vi "Hab Lifter TeleOp - PID.vi"(11 "Controller Values":T1) -> ()   [LabVIEW 2018]
uses:
  Support Code/Controller Values.ctl
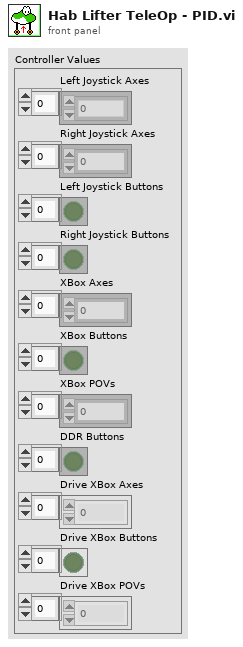
[diagram p1: front panel]
types:
  T1 = typedef "Controller Values.ctl" = cluster{"Left Joystick Axes ":dbl[], "Right Joystick Axes":dbl[], "Left Joystick Buttons":bool[], "Right Joystick Buttons":bool[], "XBox Axes":dbl[], "XBox Buttons":bool[], "XBox POVs":i16[], "DDR Buttons":bool[], "Drive XBox Axes":dbl[], "Drive XBox Buttons":bool[], "Drive XBox POVs":i16[]}
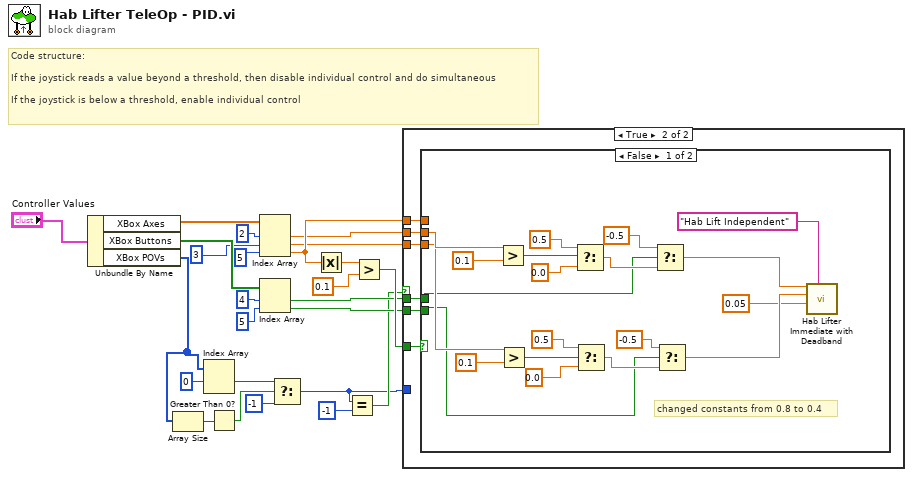
[diagram p0: block diagram]
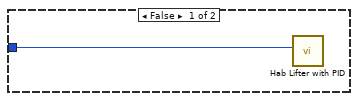
[diagram p2: hidden frame]
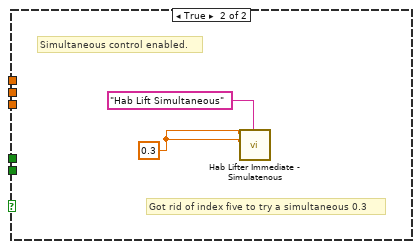
[diagram p3: hidden frame]
diagram:
  # "Code structure:\n\nIf the joystick reads a value beyond a threshold, then disable individual control and do simultaneous\n\nIf the joystick is below a threshold, enable individual control"
  n1 = Unbundle By Name("Controller Values") -> ("XBox Axes"=w24:dbl[], "XBox Buttons"=w23:bool[], "XBox POVs"=w1:i16[])
  n2 = Array Size(array=w1) -> (size(s)=w8:i32)
  n3 = Index Array(array=w1, index #1=0 ("index")) -> (element #1=w7:i16)  [unwired: 1 in, 1 out]
  n4 = Greater Than 0?(x=w8) -> (x > 0?=w9:bool)
  n5 = Index Array(array=w24, index #1=2 ("index"), index #2=3 ("index"), index #3=5 ("index")) -> (element #1=w13:dbl, element #2=w12:dbl, element #3=w14:dbl)
  n6 = Index Array(array=w23, index #1=4 ("index"), index #2=5 ("index")) -> (element #1=w11:bool, element #2=w10:bool)
  n7 = Select(t=w7, s=w9, f=i16 -1) -> (s? t:f=w2:i16)
  n8 = Absolute Value(x=w14) -> (abs(x)=w17:dbl)
  n9 = Equal?(x=w2, y=i16 -1) -> (x = y?=w3:bool)
  n10 = Greater?(x=w17, y=0.1) -> (0:w15:bool)
  n11 = case shown="True" w3 {
    tunnel: w15 -> [_ w32]
    tunnel: w14 -> [_ w31]
    tunnel: w13 -> [_ w30]
    tunnel: w12 -> [_ w29]
    tunnel: w11 -> [_ w28]
    tunnel: w10 -> [_ w27]
    tunnel: w2 -> [w26 _]
    frame False {
      n12 = call "Hab Lifter with PID.vi"("PID Position"=w26) -> ()  [unwired: 10 in, 1 out]
    }
    frame True {
      n13 = case shown="False" w32 {
        tunnel: w31 -> [_ _]
        tunnel: w30 -> [w52 _]
        tunnel: w29 -> [w50 _]
        tunnel: w28 -> [w43 _]
        tunnel: w27 -> [w37 _]
        frame False {
          # "changed constants from 0.8 to 0.4"
          n14 = Greater?(x=w52, y=0.1) -> (0:w48:bool)
          n15 = Greater?(x=w50, y=0.1) -> (0:w47:bool)
          n16 = Select(t=0.5, s=w48, f=0.0) -> (s? t:f=w46:dbl)
          n17 = Select(t=0.5, s=w47, f=0.0) -> (s? t:f=w39:dbl)
          n18 = Select(t=-0.5, s=w43, f=w46) -> (s? t:f=w36:dbl)
          n19 = Select(t=-0.5, s=w37, f=w39) -> (s? t:f=w35:dbl)
          n20 = call "Hab Lifter Immediate with Deadband.vi"("Description"="Hab Lift Independent", "Deadband Value"=0.05, "Back Setpoint"=w35, "Front Setpoint"=w36) -> ()  [unwired: 7 in, 1 out]
        }
        frame True {
          w53 = 0.3
          # "Got rid of index five to try a simultaneous 0.3"
          # "Simultaneous control enabled."
          n21 = call "Hab Lifter Immediate - Simulatenous.vi"("Description"="Hab Lift Simultaneous", "Right Setpoint"=w53, "Left Setpoint"=w53) -> ()  [unwired: 8 in, 1 out]
        }
      }
    }
  }
